vi "Calc Lift Speeds.vi"(9 "Lift Speed":dbl, 10 "Lower Limit Switch":bool, 11 "Upper Limit Switch":bool) -> (3 "Lift Speed":dbl)   [LabVIEW 2018]
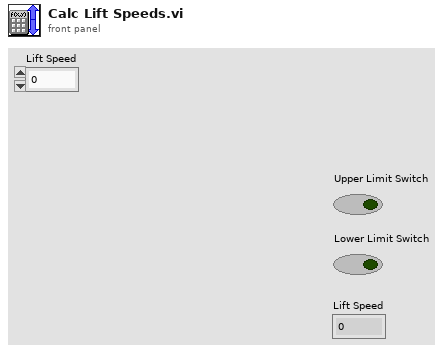
[diagram p1: front panel]
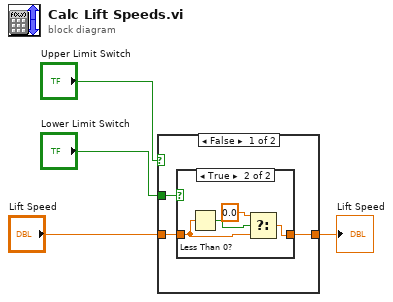
[diagram p0: block diagram]
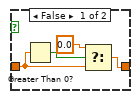
[diagram p4: hidden frame]
diagram:
  n1 = case shown="False" "Upper Limit Switch" {
    tunnel: "Lift Speed" -> [w7 w15]
    tunnel: [w6 w14] -> w3
    tunnel: "Lower Limit Switch" -> [w5 w13]
    frame False {
      n2 = case shown="True" w5 {
        tunnel: w7 -> [w8 w10]
        tunnel: [w8 w9] -> w6
        frame False {
        }
        frame True {
          n3 = Less Than 0?(x=w10) -> (x < 0?=w12:bool)
          n4 = Select(t=0.0, s=w12, f=w10) -> (s? t:f=w9:dbl)
        }
      }
    }
    frame True {
      n5 = case shown="True" w13 {
        tunnel: w15 -> [w17 w20]
        tunnel: [w16 w20] -> w14
        frame False {
          n6 = Greater Than 0?(x=w17) -> (x > 0?=w19:bool)
          n7 = Select(t=0.0, s=w19, f=w17) -> (s? t:f=w16:dbl)
        }
        frame True {
        }
      }
    }
  }
  "Lift Speed" <- w3
